vi "Run.vi"(8 "error in (no error)":errorcluster, 11 "Wavepond in":refnum<class "Wavepond.lvclass">) -> (0 "error out":errorcluster, 3 "Wavepond out":refnum<class "Wavepond.lvclass">)   [LabVIEW 2015, in "Wavepond.lvclass"]
uses:
  Wavepond.lvclass
  Wavepond Commands.ctl
  Wavepond.lvclass/Wavepond.ctl
  <vilib>/Utility/file.llb/Read From Spreadsheet File (DBL).vi
panel:
  out "size(s)":i32
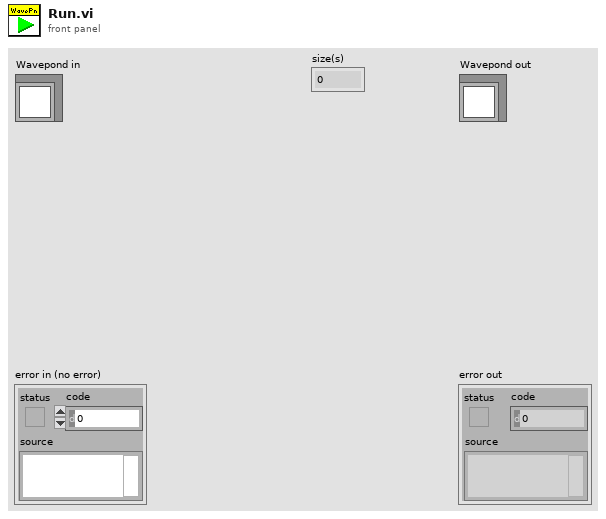
[diagram p1: front panel]
types:
  T1 = typedef "Wavepond.lvclass/Wavepond Commands.ctl" = enum16{"Initialize", "SetFrequency", "SetAtten", "WriteData", "EnableSweep", "SetLoopCnt", "SetClkDiv", "SelExtTrig", "SoftTrig", "En_SqWave"}
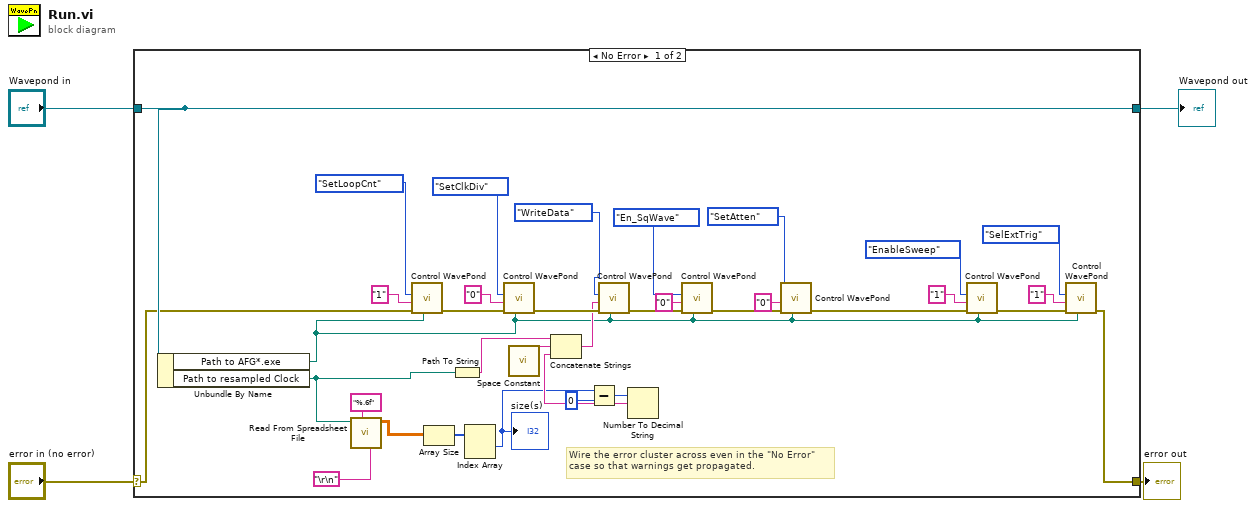
[diagram p0: block diagram]
diagram:
  n1 = case shown="No Error" "error in (no error)" {
    selector: "error in (no error)" -> [w10 w41]
    tunnel: [w28 w41] -> w3
    tunnel: [w27 w40] -> w1
    tunnel: "Wavepond in" -> [w27 w40]
    frame No Error {
      # "Wire the error cluster across even in the \"No Error\"\ncase so that warnings get propagated."
      n2 = Unbundle By Name(w27) -> ("Path to AFG*.exe"=w6:path, "Path to resampled Clock"=w24:path)
      n3 = call-poly <vilib>:"Read From Spreadsheet File.vi"("delimiter (\\t)"="\r\n", "format (%.3f)"="%.6f", "file path (dialog if empty)"=w24) -> ("all rows"=w21:dbl[][])  [unwired: 4 in, 4 out]
      n4 = call "Control WavePond.vi"("working directory"=w6, "Error In"=w10, "Parameter"="1", "Command"=Wavepond_Commands."SetLoopCnt") -> ("Error Out"=w37:errorcluster)  [unwired: 5 in, 2 out]
      n5 = Array Size(array=w21) -> (size(s)=w20:i32[])
      n6 = Path To String(path=w24) -> (string=w26:string)
      n7 = Index Array(array=w20) -> (element #1=w18:i32)  [unwired: 2 in, 1 out]
      "size(s)" <- w18
      n8 = call "Control WavePond.vi"("working directory"=w6, "Error In"=w37, "Parameter"="0", "Command"=Wavepond_Commands."SetClkDiv") -> ("Error Out"=w31:errorcluster)  [unwired: 5 in, 2 out]
      n9 = call <vilib>:"Space Constant.vi"() -> ("String"=w34:string)
      n10 = Subtract(x=w18, y=0) -> (x-y=w19:i32)
      n11 = Number To Decimal String(number=w19) -> (decimal integer string=w35:string)  [unwired: 1 in]
      n12 = Concatenate Strings(w26, w34, w35) -> (w25:string)
      n13 = call "Control WavePond.vi"("working directory"=w6, "Error In"=w31, "Parameter"=w25, "Command"=Wavepond_Commands."WriteData") -> ("Error Out"=w30:errorcluster)  [unwired: 5 in, 2 out]
      n14 = call "Control WavePond.vi"("working directory"=w6, "Error In"=w30, "Parameter"="0", "Command"=Wavepond_Commands."En_SqWave") -> ("Error Out"=w9:errorcluster)  [unwired: 5 in, 2 out]
      n15 = call "Control WavePond.vi"("working directory"=w6, "Error In"=w9, "Parameter"="0", "Command"=Wavepond_Commands."SetAtten") -> ("Error Out"=w5:errorcluster)  [unwired: 5 in, 2 out]
      n16 = call "Control WavePond.vi"("working directory"=w6, "Error In"=w5, "Parameter"="1", "Command"=Wavepond_Commands."EnableSweep") -> ("Error Out"=w32:errorcluster)  [unwired: 5 in, 2 out]
      n17 = call "Control WavePond.vi"("working directory"=w6, "Error In"=w32, "Parameter"="1", "Command"=Wavepond_Commands."SelExtTrig") -> ("Error Out"=w28:errorcluster)  [unwired: 5 in, 2 out]
    }
    frame Error {
    }
  }
  "error out" <- w3
  "Wavepond out" <- w1
